vi "Destroy to SSH.vi"(8 "Error In":errorcluster, 11 "SFTP Attributes":refnum<class "SFTP Attributes.lvclass">) -> (0 "Error Out":errorcluster, 3 "SSH":refnum<class "SSH.lvclass">)   [LabVIEW 2018, in "Toolkit.lvlib" / "SFTP Attributes.lvclass"]
doc: "Deallocates, or frees, the memory allocated for the libssh2lv shared library SFTP Attributes struct represented by this SFTP Attributes object. After this is called, the object can no longer be used in the application without causing a segmentation fault, i.e. crashing LabVIEW. This VI must be called to avoid leaking memory or running Out-of-Memory (OOM) on resource-constrained systems."
uses:
  SFTP Attributes.lvclass
  SSH/SSH.lvclass
  SFTP Attributes.lvclass/SFTP Attributes.ctl
  SSH/SSH.lvclass/SSH.ctl
  Toolkit.lvlib
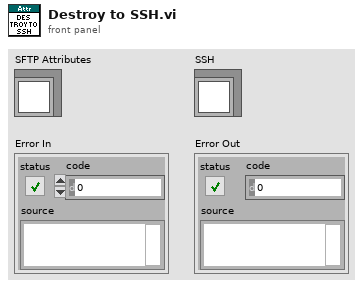
[diagram p1: front panel]
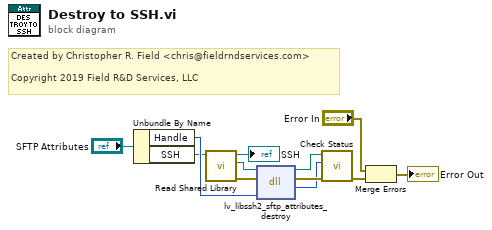
[diagram p0: block diagram]
diagram:
  # "Created by Christopher R. Field <chris@fieldrndservices.com>\n\nCopyright 2019 Field R&D Services, LLC"
  n1 = Unbundle By Name("SFTP Attributes") -> ("Handle"=w10:u64, "SSH"=w4:refnum<class "SSH.lvclass">)
  n2 = call "Read Shared Library.vi"("SSH In"=w4) -> ("Error Out"=w3:errorcluster, "libssh2lv Shared Library"=w2:path, "SSH Out"=→"SSH":refnum<class "SSH.lvclass">)  [unwired: 8 in]
  n3 = dll-call lib="lv-libssh2.*" fn="lv_libssh2_sftp_attributes_destroy"(path in=w2, error in=w3, "handle"=w10) -> (path out=w8:path, error out=w9:errorcluster, "status"=w7:i32)  [unwired: 2 in]
  n4 = call "Check Status.vi"("Error In"=w9, "Status"=w7, "libssh2lv Shared Library In"=w8) -> ("Error Out"=w6:errorcluster)  [unwired: 7 in, 1 out]
  n5 = Merge Errors("Error In", w6) -> (→"Error Out":errorcluster)
